vi "电平选择.vi"(1 "电平输入":enum16{"200mV~2V", "500mV~5V"}(ring)) -> (0 "电平输出":dbl[](array[numeric]))   [LabVIEW 2015]
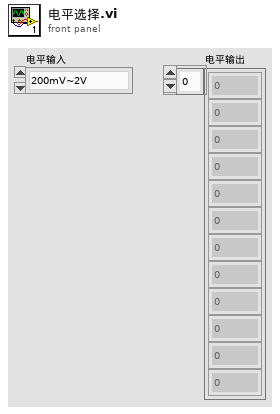
[diagram p1: front panel]
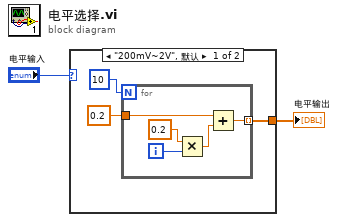
[diagram p0: block diagram]
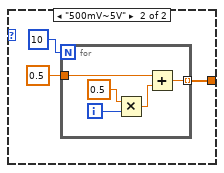
[diagram p2: hidden frame]
diagram:
  n1 = case shown="\"200mV~2V\", 默认" "电平输入" {
    tunnel: [w3 w11] -> w2
    frame "200mV~2V", Default {
      n2 = for {
        N: 10 -> [_]
        tunnel: 0.2 -> [w10]
        tunnel: [w9] -> w3 mode=indexing
        i -> [w7]
        n3 = Multiply(x=0.2, y=w7) -> (x*y=w6:dbl)
        n4 = Add(x=w10, y=w6) -> (x+y=w9:dbl)
      }
    }
    frame "500mV~5V" {
      n5 = for {
        N: 10 -> [_]
        tunnel: 0.5 -> [w18]
        tunnel: [w17] -> w11 mode=indexing
        i -> [w15]
        n6 = Multiply(x=0.5, y=w15) -> (x*y=w14:dbl)
        n7 = Add(x=w18, y=w14) -> (x+y=w17:dbl)
      }
    }
  }
  "电平输出" <- w2
